vi "Eval_SglVar.vi"(8 "error in (no error)":errorcluster, 10 "varValue":dbl format="%#_13g", 11 "muExpr in":refnum<class "mupExpr.lvclass">) -> (0 "error out":errorcluster, 2 "Result":dbl, 3 "muExpr out":refnum<class "mupExpr.lvclass">)   [LabVIEW 2015, in "mupExpr.lvclass"]
uses:
  mupExpr.lvclass
  mupExpr.lvclass/mupExpr.ctl
  mupLib/mupEval.vi
  mupLib/mupCheckError.vi
  mupLib/mupLibPath.vi
  mupLib/mupLib.lvlib
panel:
  # "Update the value of the \"Single Variable\" then evaluate the expression"
  # "If the expression contains no variables, the valuie is ignored.\n\nIf the expression contains more than one variable and no variable has been selected as the \"single variable\"\nan error will be generated."
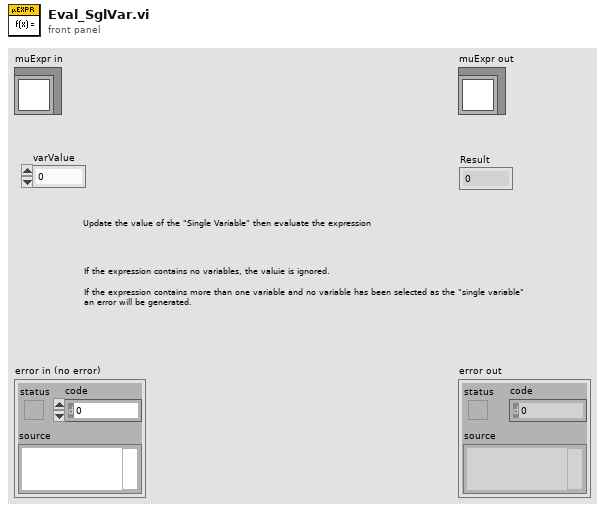
[diagram p1: front panel]
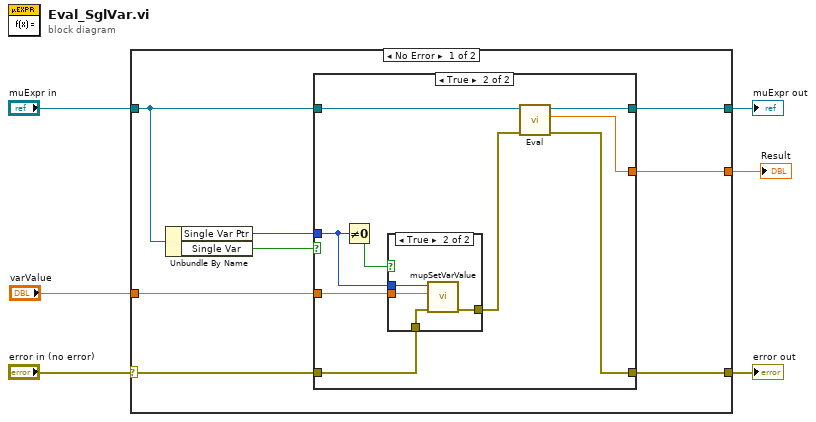
[diagram p0: block diagram]
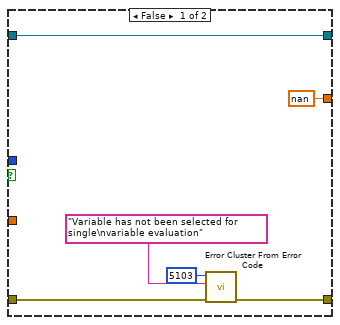
[diagram p2: hidden frame]
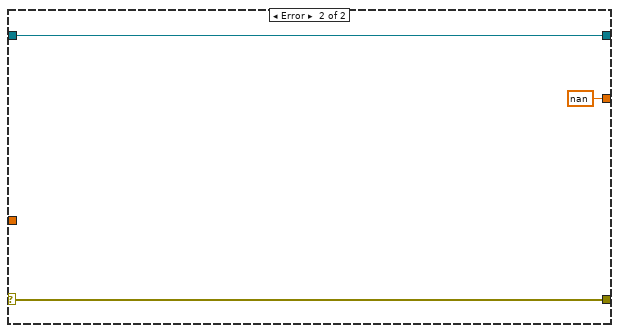
[diagram p4: hidden frame]
diagram:
  n1 = case shown="No Error" "error in (no error)" {
    selector: "error in (no error)" -> [w13 w37]
    tunnel: [w8 w37] -> w5
    tunnel: [w9 w36] -> w3
    tunnel: "muExpr in" -> [w12 w36]
    tunnel: "varValue" -> [w10 _]
    tunnel: [w7 nan ("Result")] -> w1
    frame No Error {
      n2 = Unbundle By Name(w12) -> ("Single Var Ptr"=w11:u64, "Single Var"=w14:bool)
      n3 = case shown="True" w14 {
        tunnel: w13 -> [w20 w29]
        tunnel: w12 -> [w16 w26]
        tunnel: w11 -> [_ w22]
        tunnel: w10 -> [_ w28]
        tunnel: [w16 w25] -> w9
        tunnel: [w19 w24] -> w8
        tunnel: [nan ("Result") w23] -> w7
        frame False {
          n4 = call <vilib>:"Error Cluster From Error Code.vi"("error in (no error)"=w20, "error message (\"\")"="Variable has not been selected for single\nvariable evaluation" ("error message (\"\")"), "error code (0)"=5103) -> ("error out"=w19:errorcluster)  [unwired: 6 in]
        }
        frame True {
          n5 = Not Equal To 0?(x=w22) -> (x != 0?=w21:bool)
          n6 = case shown="True" w21 {
            tunnel: w29 -> [w30 w34]
            tunnel: w28 -> [_ w32]
            tunnel: [w30 w33] -> w27
            tunnel: w22 -> [_ w31]
            frame False {
            }
            frame True {
              n7 = call "mupSetVarValue.vi"("error in (no error)"=w34, "varValue"=w32, "varPtr in"=w31) -> ("error out"=w33:errorcluster)  [unwired: 7 in, 1 out]
            }
          }
          n8 = call "Eval.vi"("error in (no error)"=w27, "muExpr in"=w26) -> ("error out"=w24:errorcluster, "Result"=w23:dbl, "muExpr out"=w25:refnum<class "mupExpr.lvclass">)  [unwired: 7 in]
        }
      }
    }
    frame Error {
    }
  }
  "error out" <- w5
  "muExpr out" <- w3
  "Result" <- w1
